vi "Stoic_Mean_Calc.vi"() -> ()   [LabVIEW 2014]
uses:
  <vilib>/Analysis/baseanly.llb/Mean (DBL).vi
  <vilib>/Utility/file.llb/Read From Spreadsheet File (DBL).vi
  <vilib>/Analysis/NI_AALBase.lvlib
panel:
  in  "Test Vi":bool
  out "Mean":dbl format="%0.2f"
  out "Mean Array":dbl[](array[numeric])
  out "Min value":dbl
  out "Max value":dbl
  in  "Cycle Length":dbl
  out "20% Bin Index":i32[](array[numeric])
  out "Bin Array":dbl[](array[numeric])
  out "Temp Values":dbl[](array[numeric])
  in  "file path (dialog if empty)":path
  out "Max Bin":dbl
  out "Min Bin":dbl
  in  "Multiple":dbl
  in  "Array In":dbl[](array[numeric])
  # "Stoic Temperature Mean"
  # "Overall"
  # "Stoic"
  # "(Used for Testing)"
  # "For Testing VI:\nUse Tab delimited file from excel with all data Transposed\nto the top Row.\nOpen Vi in Windows not RT."
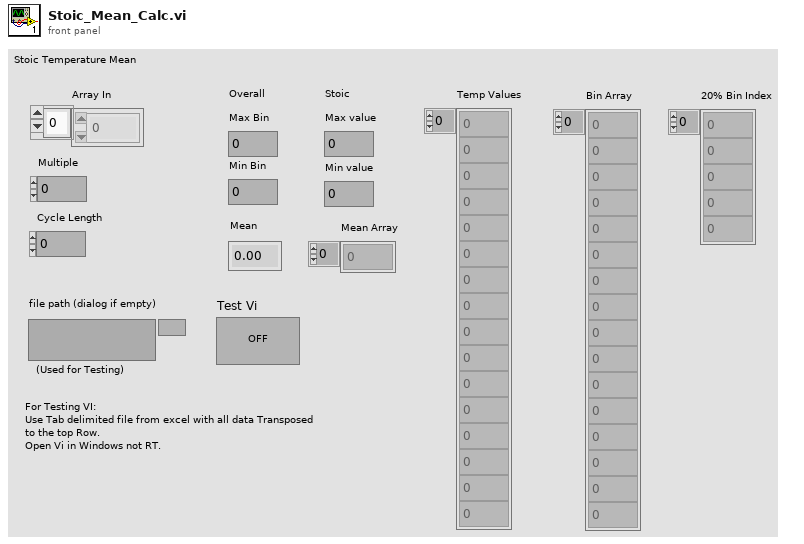
[diagram p1: front panel]
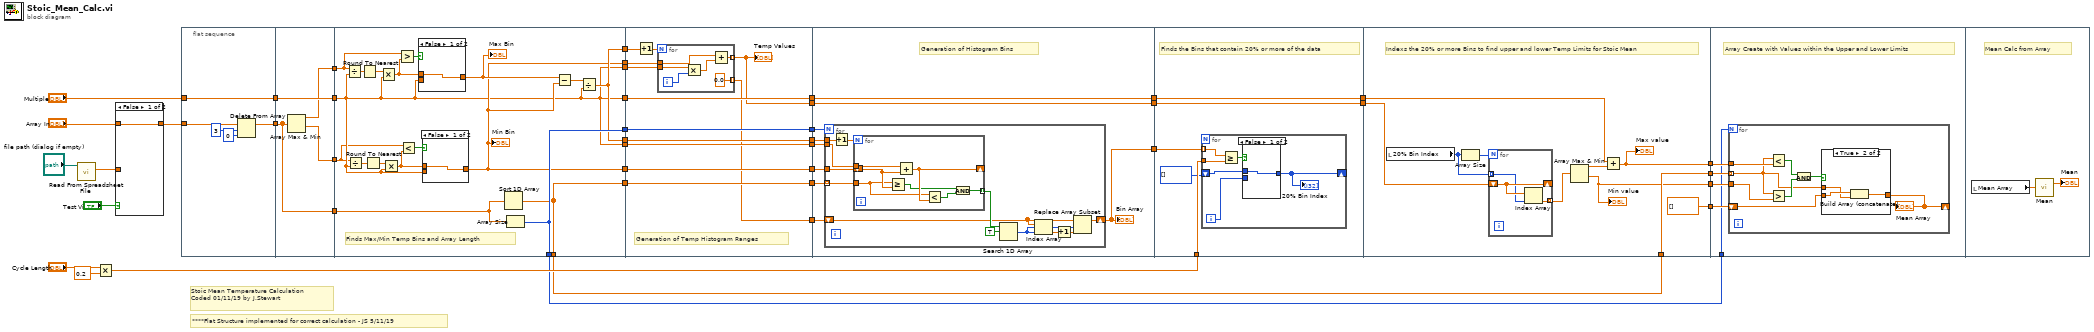
[diagram p0: block diagram]
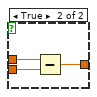
[diagram p3: hidden frame]
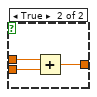
[diagram p4: hidden frame]
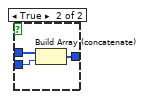
[diagram p5: hidden frame]
diagram:
  # "****Flat Structure implemented for correct calculation - JS 5/11/19"
  # "Stoic Mean Temperature Calculation\nCoded 01/11/19 by J.Stewart"
  n1 = call-poly <vilib>:"Read From Spreadsheet File.vi"("file path (dialog if empty)"="file path (dialog if empty)") -> ("first row"=w40:dbl[])  [unwired: 6 in, 4 out]
  n2 = Multiply(x="Cycle Length", y=0.2) -> (x*y=w33:dbl)
  n3 = case shown="False" "Test Vi" {
    tunnel: w40 -> [_ w45]
    tunnel: [w44 w45] -> w1
    tunnel: "Array In" -> [w44 _]
    frame False {
    }
    frame True {
    }
  }
  n4 = flat-sequence {
    tunnel: "Multiple" -> [w50]
    tunnel: [w50] -> w3
    tunnel: [w47] -> w2
    tunnel: w1 -> [w46]
    tunnel: [w54] -> w7
    tunnel: [w51] -> w6
    tunnel: [w53] -> w5
    tunnel: [w52] -> w4
    tunnel: w3 -> [w54]
    tunnel: w2 -> [w51]
    tunnel: [w70] -> w18
    tunnel: [w61] -> w17
    tunnel: [w56] -> w16
    tunnel: [w69] -> w15
    tunnel: [w71] -> w14
    tunnel: [w56] -> w13
    tunnel: [w69] -> w12
    tunnel: [w61] -> w11
    tunnel: [w71] -> w10
    tunnel: [w70] -> w9
    tunnel: [w56] -> w8
    tunnel: w7 -> [w56]
    tunnel: w6 -> [w72]
    tunnel: w5 -> [w62]
    tunnel: w4 -> [w55]
    tunnel: [w85] -> w31
    tunnel: [w92] -> w30
    tunnel: [w91] -> w29
    tunnel: [w90] -> w28
    tunnel: [w89] -> w27
    tunnel: [w88] -> w26
    tunnel: [w81] -> w24
    tunnel: [w87] -> w21
    tunnel: w18 -> [w92]
    tunnel: w17 -> [w91]
    tunnel: w16 -> [w90]
    tunnel: w15 -> [w89]
    tunnel: w14 -> [w88]
    tunnel: w13 -> [w87]
    tunnel: w12 -> [w84]
    tunnel: w11 -> [w82]
    tunnel: w8 -> [w83]
    tunnel: [w107] -> w32
    tunnel: w31 -> [w106]
    tunnel: w30 -> [w105]
    tunnel: w29 -> [w104]
    tunnel: w28 -> [w103]
    tunnel: w27 -> [w102]
    tunnel: w26 -> [w101]
    tunnel: w24 -> [w100]
    tunnel: [w100] -> w23
    tunnel: w21 -> [w99]
    tunnel: [w99] -> w20
    tunnel: w33 -> [w130]
    tunnel: w32 -> [w131]
    tunnel: [w128] -> w25
    tunnel: w23 -> [w128]
    tunnel: [w127] -> w22
    tunnel: w20 -> [w127]
    tunnel: w9 -> [w151]
    tunnel: [w146] -> w37
    tunnel: [dbl[] [] ("Array 3")] -> w36
    tunnel: [w151] -> w35
    tunnel: [w145] -> w34
    tunnel: w25 -> [w143]
    tunnel: w22 -> [w142]
    tunnel: w37 -> [w158]
    tunnel: w36 -> [w157]
    tunnel: w35 -> [w156]
    tunnel: w34 -> [w159]
    tunnel: w10 -> [w155]
    frame #0 {
      n5 = Delete From Array(array=w46, length=3, index=0) -> (array with subset deleted=w47:dbl[])  [unwired: 1 out]
    }
    frame #1 {
      n6 = Array Max & Min(array=w51) -> (max value=w53:dbl, min value=w52:dbl)  [unwired: 2 out]
    }
    frame #2 {
      # "Finds Max/Min Temp Bins and Array Length"
      n7 = Divide(x=w62, y=w56) -> (x/y=w63:dbl)
      n8 = Divide(x=w55, y=w56) -> (x/y=w57:dbl)
      n9 = Round To Nearest(number=w63) -> (nearest integer value=w64:dbl)
      n10 = Round To Nearest(number=w57) -> (nearest integer value=w58:dbl)
      n11 = Multiply(x=w64, y=w56) -> (x*y=w65:dbl)
      n12 = Multiply(x=w58, y=w56) -> (x*y=w59:dbl)
      n13 = Greater?(x=w62, y=w65) -> (0:w66:bool)
      n14 = Less?(x=w55, y=w59) -> (x < y?=w60:bool)
      n15 = case shown="False" w66 {
        tunnel: w65 -> [w77 w80]
        tunnel: w56 -> [_ w79]
        tunnel: [w77 w78] -> w67
        frame False {
        }
        frame True {
          n16 = Add(x=w80, y=w79) -> (x+y=w78:dbl)
        }
      }
      "Max Bin" <- w67
      n17 = case shown="False" w60 {
        tunnel: w59 -> [w73 w76]
        tunnel: w56 -> [_ w75]
        tunnel: [w73 w74] -> w61
        frame False {
        }
        frame True {
          n18 = Subtract(x=w76, y=w75) -> (x-y=w74:dbl)
        }
      }
      "Min Bin" <- w61
      n19 = Sort 1D Array(array=w72) -> (sorted array=w70:dbl[])
      n20 = Array Size(array=w72) -> (size(s)=w71:i32)
      n21 = Subtract(x=w67, y=w61) -> (x-y=w68:dbl)
      n22 = Divide(x=w68, y=w56) -> (x/y=w69:dbl)
    }
    frame #3 {
      # "Generation of Temp Histogram Ranges"
      n23 = Increment(x=w84) -> (x+1=w86:dbl)
      n24 = for {
        N: w86 -> [_]
        tunnel: w83 -> [w98]
        tunnel: w82 -> [w97]
        tunnel: [w95] -> w81 mode=indexing
        tunnel: [0.0 ("x+y")] -> w85 mode=indexing
        i -> [w94]
        n25 = Multiply(x=w98, y=w94) -> (x*y=w96:dbl)
        n26 = Add(x=w97, y=w96) -> (x+y=w95:dbl)
      }
      "Temp Values" <- w81
    }
    frame #4 {
      # "Generation of Histogram Bins"
      n27 = for {
        N: w101 -> [_]
        tunnel: w103 -> [w118]
        tunnel: w105 -> [w119] mode=indexing
        tunnel: w102 -> [w108]
        tunnel: w104 -> [w117]
        shift-right: [w116] -> w107
        shift-left: w106 -> [w112]
        n28 = Increment(x=w108) -> (x+1=w109:dbl)
        n29 = for {
          N: w109 -> [_]
          tunnel: w119 -> [w122]
          tunnel: w118 -> [w120]
          shift-right: [w125] -> _
          shift-left: w117 -> [w126]
          tunnel: [w121] -> w115 mode=indexing
          n30 = Greater Or Equal?(x=w122, y=w126) -> (x >= y?=w123:bool)
          n31 = Add(x=w120, y=w126) -> (x+y=w125:dbl)
          n32 = Less?(x=w122, y=w125) -> (x < y?=w124:bool)
          n33 = And(x=w123, y=w124) -> (x .and. y?=w121:bool)
        }
        n34 = Search 1D Array(1D array=w115, element=TRUE) -> (index of element=w113:i32)  [unwired: 1 in]
        n35 = Index Array(array=w112, index=w113) -> (element=w111:dbl)
        n36 = Increment(x=w111) -> (x+1=w110:dbl)
        n37 = Replace Array Subset(array=w112, new element=w110, index=w113) -> (w116:dbl[])
      }
      "Bin Array" <- w107
    }
    frame #5 {
      # "Finds the Bins that contain 20% or more of the data"
      n38 = for {
        tunnel: w131 -> [w137] mode=indexing
        shift-right: [w134] -> _
        shift-left: i32[] [] -> [w133]
        tunnel: w130 -> [w132]
        i -> [w135]
        n39 = Greater Or Equal?(x=w137, y=w132) -> (x >= y?=w136:bool)
        n40 = case shown="False" w136 {
          tunnel: w135 -> [_ w141]
          tunnel: [w138 w140] -> w134
          tunnel: w133 -> [w138 w139]
          frame False {
          }
          frame True {
            n41 = Build Array (concatenate)(w139, w141) -> (w140:i32[])
          }
        }
        "20% Bin Index" <- w134
      }
    }
    frame #6 {
      # "Indexs the 20% or more Bins to find upper and lower Temp Limits for Stoic Mean"
      n42 = local read "20% Bin Index"() -> (w144:i32[])
      n43 = Array Size(array=w144) -> (size(s)=w147:i32)
      n44 = for {
        N: w147 -> [_]
        tunnel: w144 -> [w153] mode=indexing
        shift-right: [w154] -> _
        shift-left: w143 -> [w154]
        tunnel: [w152] -> w148 mode=indexing
        n45 = Index Array(array=w154, index=w153) -> (element=w152:dbl)
      }
      n46 = Array Max & Min(array=w148) -> (max value=w149:dbl, min value=w145:dbl)  [unwired: 2 out]
      "Min value" <- w145
      n47 = Add(x=w142, y=w149) -> (x+y=w146:dbl)
      "Max value" <- w146
    }
    frame #7 {
      # "Array Create with Values within the Upper and Lower Limits"
      n48 = for {
        N: w155 -> [_]
        tunnel: w159 -> [w167]
        tunnel: w158 -> [w166]
        shift-right: [w160] -> _
        shift-left: w157 -> [w162]
        tunnel: w156 -> [w161] mode=indexing
        n49 = Less?(x=w161, y=w166) -> (x < y?=w165:bool)
        n50 = Greater?(x=w161, y=w167) -> (0:w164:bool)
        n51 = And(x=w165, y=w164) -> (x .and. y?=w163:bool)
        n52 = case shown="True" w163 {
          tunnel: w162 -> [w168 w171]
          tunnel: [w168 w170] -> w160
          tunnel: w161 -> [_ w169]
          frame False {
          }
          frame True {
            n53 = Build Array (concatenate)(w171, w169) -> (w170:dbl[])
          }
        }
        "Mean Array" <- w160
      }
    }
    frame #8 {
      # "Mean Calc from Array"
      n54 = local read "Mean Array"() -> (w173:dbl[])
      n55 = call-poly <vilib>:"Mean.vi"("X"=w173) -> ("mean"=→"Mean":dbl)  [unwired: 1 out]
    }
  }
